vi "AlliGator Menu Items.vi"(8 "Error In":errorcluster, 9 "Menu Item Tag":string, 11 "This VI":refnum<vi>) -> (0 "Error Out":errorcluster, 1 "Message":string, 2 "Window opened?":bool, 3 "AlliGator Actions":T1[](array[typedef]))   [LabVIEW 2021, in "AlliGator GUI.lvlib"]
doc: "Handles AlliGator menu items that are always responsive, including when AlliGator is busy."
uses:
  AlliGator GUI.lvlib
  Action Engine/AlliGator Q Element.ctl
  Action Engine/AlliGator Q Event.ctl
  AlliGator Windows List.ctl
  AlliGator Open Wndow Event Data.ctl
  GUI/Open VI Options.ctl
  Globals, Variables, Constants/AlliGator Variables List.ctl
  Intensity Corrections/AlliGator Define & Save Intensity Corrections File.vi
  Variant/Variant to Data/Variant to Boolean.vi
  Globals, Variables, Constants/AlliGator Abort.vi
  AlliGator Check Version.vi
  <vilib>/Platform/browser.llb/Open URL in Default Browser (string).vi
  Utilities/Utilities.lvlib
  Intensity Corrections/AlliGator Intensity Corrections.lvlib
  Settings/AlliGator Settings.lvlib
  Globals, Variables, Constants/AlliGator Globals, Variables & Constants.lvlib
  Variant/Variant to Data/Variant to Data.lvlib
  Action Engine/AlliGator Action Engine.lvlib
  GUI/GUI.lvlib
panel:
  # "see the AlliGator License on the block diagram (Ctrl+E or Window:Show Block Diagram)"
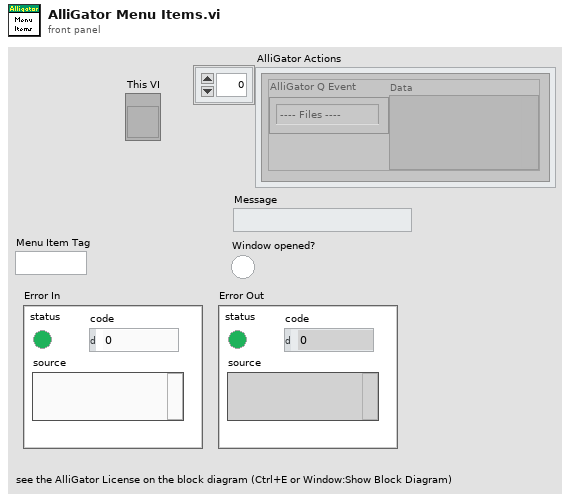
[diagram p1: front panel]
types:
  T1 = typedef "AlliGator Action Engine.lvlib/AlliGator Q Element.ctl" = cluster{"AlliGator Q Event":T2, "Data":variant}
  T2 = typedef "AlliGator Action Engine.lvlib/AlliGator Q Event.ctl" = enum16{"---- Files ----", "Files:Set Batch Export Files To Save", "Files:Set Dataset Loading & Pre-processing Options", "Files:Check #Frames in Dataset", "Files:Increment Frame Index", "Files:Open Mask Image", "Files:Open White Light Image", "Files:Open Single Dataset", "Files:New Folder of Folders Selected", "Files:Load File (all Types)_Scriptable", "Files:Move Flattened Series to Folders Series", "Files:Select Folder", "Files:Load FLI Dataset", "Files:Load Swiss SPAD 1 Dataset", "Files:Load Swiss SPAD 2 Dataset", "Files:Load .sdt FLI Dataset", "Files:Load .ptu FLI Dataset", "Files:Load .bin FLI Dataset", "Files:Load Single Gate Image Folder", "Files:Load I/m/phi Dataset (deprecated)", "Files:Load Single Image", "Files:Subtract Background File", "Files:Export FLI Dataset", "Files:Load HDF5 FLI Dataset", "Files:Set Destination File Path", "Files:Save Mask Image", "Files:Batch Conversion", "Files:New Folder Selected", "Files:Close FLI Dataset", "Files:Close FLI Dataset Series", "Files:Close White Light Image", "Files:Close Mask Image", "---- FLI Dataset ----", "FLI Dataset:Channel Arithmetic", "FLI Dataset:Export Average Lifetime Map as ASCII", "FLI Dataset:Export User-Defined Quantity Map as ASCII", "FLI Dataset:Python Function FLI Dataset Event", "FLI Dataset:ROI Analysis", "FLI Dataset:Tilted Logistic Square Gated IRF Characteristics Map", "FLI Dataset:Logistic Square Gated IRF Characteristics Map", "FLI Dataset:Square Gated IRF Characteristics Map", "FLI Dataset:Multi-ROI Single-Pixel Phasor Analysis", "FLI Dataset:Multi-ROI Single-Pixel NLSF Analysis", "FLI Dataset:All ROIs IRF Extraction", "FLI Dataset:All ROIs Decay Fit Non-Interactive (Fast + Individual IRF)", "FLI Dataset:All ROIs Phasor Analysis", "FLI Dataset:All ROIs Decay Fit", "FLI Dataset:Fluorescence Decay Statistics", "FLI Dataset:Update Decay Statistics Graph", "FLI Dataset:Get Decay from ROI", "FLI Dataset:All ROIs Average Lifetimes", "---- FLI Dataset Series ----", "FLI Dataset Series:Sum All Datasets in Series", "FLI Dataset Series:Add Dataset to Accumulated Dataset", "FLI Dataset Series:Display Accumulated Dataset", "FLI Dataset Series:Clear Dataset Series Sum", "FLI Dataset Series:Time-Series Analysis (NLSF)", "FLI Dataset Series:Time-Series Analysis (Phasor)", "---- Image ----", "Image:Update Image Profile Plots", "Image:Image Histogram Cursor Move", "Image:Image Histogram", "Image:Image Contrast", "Image:Set Image Histogram Cursor Move Flag", "Image:Clear Image Overlay", "Image:Use ROI as Search Area", "Image:Set ROI Diameter", "Image:Save Image Data as TIFF", "Image:Save Displayed Image with Overlay", "Image:Save Image Overlay Only", "Image:Save Image as Hot Pixel Mask", "Image:Change Source Image Color Palette", "Image:Copy Image to Clipboard", "Image:Source Image ROI Selection", "Image:Delete All ROIs", "Image:Delete All Unselected ROIs", "Image:Delete ROI", "Image:Merge All ROIs", "Image:Store ROI", "Image:Source Image ROI Storage", "Image:Export ROI Description to Notebook", "Image:Save ROI", "Image:Load ROI", "Image:Paste ROI Definition", "Image:Clear ROI", "Image:Identify ROIs in Mask Image", "Image:Create Complementary ROI", "Image:Create Contour ROI", "Image:Create ROI(s) from Pixels with Peak above Min_Scriptable", "Image:Create ROI(s) from Pixels with Intensity above Min_Scriptable", "Image:Compute ROI Statistics", "Image:Delete ROI(s) based on ROI Characteristics", "Image:Create ROI Grid", "Image:ROI to Individual Pixel ROIs", "Image:Python Function Source Image Event", "Image:Show Phasor Calibration Map ROI Centers", "Image:Convert ROI to Mask Image", "Image:Mouse Move", "Image:Mouse Up", "Image:Set Source Image Mouse Move Flag", "Image:Add Scale Bar Overlay", "Image:Delete Existing ROIs Option", "Image:Overlay ROI Median", "Image:Check Current ROI", "---- Decay ----", "Decay:Clear IRF/Reference Plot", "Decay:Clear Local IRFs", "Decay:Add Decay to Graph", "Decay:Smoothen Plot", "Decay:Smoothen Plot Tail", "Decay:Average Selected Plots", "Decay:Extract IRF", "Decay:Optimal IRF Extraction", "Decay:Threshold IRF", "Decay:Fit to Model IRF", "Decay:Fit IRF to Square Gate", "Decay:Fit IRF to Logistic Square Gate", "Decay:Fit IRF to Tilted Logistic Square Gate", "Decay:Create Bounding Cursors Set", "Decay:Export Bounding Cursors Definition to Notebook", "Decay:Denoise Plot", "Decay:Compute Cumulative Function", "Decay:Use as Reference Decay", "Decay:Show Reference Decay/IRF", "Decay:Extrapolate Decay", "Decay:Create Head & Tail Bounding Cursors", "Decay:Store Cursor-defined Head & Tail Fractions", "Decay:Rebin Plot", "Decay:1-Normalize Decay", "Decay:[0-1]-Normalize Plot", "Decay:Straighten Decay", "Decay:Shift Decay", "Decay:Fold Decay", "Decay:Fit Decay", "Decay:Global Fit of Selected Decays", "Decay:Post Global Fit Script", "Decay:Add Global Fit Parameters to Graph", "Decay:Add Decay Parameter(s) to Plot (Graph)", "Decay:Export Decay to Phasor Graph", "Decay:Plot Decay Shifts", "Decay:Compute Average Lifetime", "Decay:Plot Convolution", "Decay:Graph Tip Strip Update", "---- Decay Statistics ----", "Decay Statistics:Tip Strip Update", "---- Intensity Time Trace ----", "Intensity Time Trace:Use File Timestamp", "Intensity Time Trace:Load Intensity Corrections File", "Intensity Time Trace:Clear Intensity Corrections File", "Intensity Time Trace:Tip Strip Update", "---- Phasor Plot ----", "Phasor Plot:Build Phasor Plot", "Phasor Plot:Change Phasor Plot Color Palette", "Phasor Plot:Adjust Phasor Plot Display Range", "Phasor Plot:Highlight Image ROI in Phasor Plot", "Phasor Plot:Save Phasor Plot Image with Overlay", "Phasor Plot:Export Complex Phasor Map", "Phasor Plot:Export Phasor Ratio Map", "Phasor Plot:Export Average Lifetime Map", "Phasor Plot:Compute Phase Lifetime Histogram", "Phasor Plot:Compute Phasor Ratio Histogram", "Phasor Plot:Compute Phase Lifetime vs Intensity Scatter Plot", "Phasor Plot:Weber 2-Component Decomposition", "Phasor Plot:Update Phasor Color Map Vertices", "Phasor Plot:Clear Phasor Overlay", "Phasor Plot:Use Segment Extremities as References", "Phasor Plot:Use UC/Segment Intersections as References", "Phasor Plot:Use UC/Principal Axis Intersections as References", "Phasor Plot:Use UC/Linear Fit Intersections as References", "Phasor Plot:Update Phasor Plot Reference", "Phasor Plot:Show Local Phasor Info in Phasor Plot", "Phasor Plot:Update Phasor Plot State", "Phasor Plot:Phasor Plot ROI Storage", "Phasor Plot:Phasor Plot ROI Selection", "Phasor Plot:Python Function Phasor Plot Event", "Phasor Plot:Overlay Phasor ROI, Ratio or Map in Source Image", "Phasor Plot:Compute Decay of Selected Phasors", "Phasor Plot:Phasor at Image Pixel", "Phasor Plot:Mouse Move", "Phasor Plot:Mouse Up", "Phasor Plot:Display Range Mouse Move", "Phasor Plot:Set Mouse Move Flag", "---- Phasor Graph ----", "Phasor Graph:Calibrated Phasor Map Series", "Phasor Graph:Whole Image Phasor Scatter Plot (deprecated)", "Phasor Graph:Get Phasor Value", "Phasor Graph:Create New Phasor Plot Dialog", "Phasor Graph:Update Last Phasor Value", "Phasor Graph:Update Phasor (m, phi)", "Phasor Graph:Remove Single Phasor from Plot", "Phasor Graph:Add Single Phasor to Plot", "Phasor Graph:Remove Phasor Plot", "Phasor Graph:Remove Selected Phasor Plots", "Phasor Graph:Clear Phasor Data", "Phasor Graph:Clear Phasor Graph", "Phasor Graph:Cursor Move", "Phasor Graph:Draw Cursor Connecting Line", "Phasor Graph:Clear Cursor Connecting Line", "Phasor Graph:Find UC Intersection", "Phasor Graph:Use UC/Cursor-Defined Line Intersections", "Phasor Graph:Use Selected Plots Fitted Line/UC Intersections", "Phasor Graph:Use Selected Plots Principal Axis/UC Intersections", "Phasor Graph:Show Single Phasor", "Phasor Graph:Save Single Phasor Plot", "Phasor Graph:Save All Phasor Plots", "Phasor Graph:Load Phasor Plot(s)", "Phasor Graph:Phasor Multiplication", "Phasor Graph:Compute Average Phasor", "Phasor Graph:Compute Multiple Average Phasors (Selected Plots)", "Phasor Graph:Export Single Phasor Plot Phase Lifetimes", "Phasor Graph:Phase Lifetime Trajectory", "Phasor Graph:Phase Lifetime vs Intensity Scatter Plot (deprecated)", "Phasor Graph:Parameter 2 vs Parameter 1 Scatter Plot", "Phasor Graph:Use Cursor n Location", "Phasor Graph:Set Reference n to Current Phase Lifetime Value", "Phasor Graph:Set Reference n to Lifetime Value", "Phasor Graph:Set Cursor n Location", "Phasor Graph:Save Phasor Graph Image", "Phasor Graph:Update SEPL Plot", "Phasor Graph:Export Single Phasor Plot Data", "Phasor Graph:Export Selected Phasor Plots Data", "Phasor Graph:Python Function Phasor Graph Event", "Phasor Graph:Tip Strip Update", "---- Calibration ----", "Calibration:Set Calibration Type", "Calibration:Load/Save Phasor Calibration", "Calibration:Load/Save Phasor Calibration Series", "Calibration:Load/Save Phasor Calibration Map", "Calibration:Use as Calibration", "Calibration:Compute Optimal Calibration from Phasor References", "Calibration:Clear Phasor Calibration", "Calibration:Single Phasor Calibration Information", "Calibration:Use as Calibration Series", "Calibration:Use as Calibration Map", "Calibration:Clear Calibration Series", "Calibration:Phasor Calibration Series Information", "Calibration:Clear Calibration Map", "Calibration:Phasor Calibration Map Information", "Calibration:Apply Phasor Calibration", "Calibration:Update Single Plot Calibration", "Calibration:Update Multiple Plots Calibration", "Calibration:Clear Single Plot Calibration", "Calibration:Clear All Plots Calibrations", "Calibration:Clear Plot(s) Calibration(s)?", "Calibration:Phasor Calibration Maps (# Gates Series)", "---- Phasor Ratio ----", "Phasor Ratio:Clear Reference n", "Phasor Ratio:Toggle Selected Plot(s)  Lock to Reference 1", "Phasor Ratio:Use as Reference n", "Phasor Ratio:Send Reference n to Notebook", "Phasor Ratio:Toggle Selected Plot(s)  Lock to Reference 2", "Phasor Ratio:Compute Phasor Ratio at Mouse Location", "Phasor Ratio:Compute Phasor Plot's Average Phasor Ratio", "Phasor Ratio:Compute Time-Series Phasor Ratios", "Phasor Ratio:Fit Line to Phasor Ratio Plot", "Phasor Ratio:Save References", "Phasor Ratio:Load References", "Phasor Ratio:Update Phasor Reference 1", "Phasor Ratio:Update Phasor Reference 2", "Phasor Ratio:Move Cursor n to Reference n", "Phasor Ratio:Use as Phasor Reference 1 Lifetime", "Phasor Ratio:Use as Phasor Reference 2 Lifetime", "Phasor Ratio:Export Phasor Ratio Map as ASCII", "Phasor Ratio:Tip Strip Update", "---- Lifetime & Other Parameters Graph ----", "Lifetime:Tip Strip Update", "---- Decay Fit Parameter Map ----", "Decay Fit Parameter Map:Export ROI NLSF Data as ASCII", "Decay Fit Parameter Map:Set Decay Fit Parameter Map Selection", "Decay Fit Parameter Map:Build Decay Fit Parameter Map", "Decay Fit Parameter Map:Change Decay Fit Parameter Map Color Palette", "Decay Fit Parameter Map:Export Decay Fit Parameter Map Data as ASCII", "Decay Fit Parameter Map:Export All Decay Fit Parameter Maps Data as ASCII", "Decay Fit Parameter Map:Selected Parameter Scatterplot", "Decay Fit Parameter Map:Parameter 2 vs Parameter 1 Scatterplot", "Decay Fit Parameter Map:Save Decay Fit Parameter Map Image", "Decay Fit Parameter Map:Save-Load IRFs & Fit Data", "Decay Fit Parameter Map:Update Local Decay Plots", "Decay Fit Parameter Map:Python Function Decay Fit Parameters Map Event", "Decay Fit Parameter Map:Overlay Decay Fit Parameter Map in Source Image", "Decay Fit Parameter Map:Selected Parameter vs Intensity Scatterplot", "Decay Fit Parameter Map:Mouse Up", "Decay Fit Parameter Map:Display Range Mouse Move", "---- Parameter Map ----", "Parameter Map:Export ROI Parameters Data as ASCII", "Parameter Map:Delete Parameter Map Set", "Parameter Map:Update Parameter List", "Parameter Map:Build Parameter Map", "Parameter Map:Change Parameter Map Color Palette", "Parameter Map:Export Parameter Map Data as ASCII", "Parameter Map:Export All Parameter Maps Data as ASCII", "Parameter Map:Selected Parameter Scatterplot", "Parameter Map:Parameter 2 vs Parameter 1 Scatterplot", "Parameter Map:Selected Parameter vs Intensity Scatterplot", "Parameter Map:Save Parameter Map Image", "Parameter Map:Save-Load IRFs & Parameter Maps (TODO)", "Parameter Map:Set Parameter Map Selection", "Parameter Map:Python Function Parameter Map Event", "Parameter Map:Overlay Parameter Map in Source Image", "Parameter Map:Update Local Decay Plots", "Parameter Map:Mouse Up", "Parameter Map:Display Range Mouse Move", "---- Generic Graph ----", "Generic Graph:Generic XY Graph Event", "Generic Graph:Python Function XY Graph Event", "Generic Graph:New Plot", "Generic Graph:Save Plot", "Generic Graph:XY Plot Histogram", "Generic Graph:Set XY Graph Plot Name", "Generic Graph:Set Last Cursor Style", "Generic Graph:Tip Strip Update", "---- GUI ----", "GUI:Start Script", "GUI:Type of Displayed Image Changed", "GUI:Gate Image Slide Changed", "GUI:Show Busy Icon", "GUI:Show Busy Icon & Abort Button", "GUI:Hide Busy Icon", "GUI:Hide Busy Icon & Abort Button", "GUI:Abort", "GUI:End Script", "GUI:Start Timing", "GUI:End Timing", "GUI:Set State Indicator", "GUI:Send Parameters JSON Strings to Clipboard", "GUI:Set Gate Step", "GUI:Idle", "GUI:Initialization", "GUI:Quit", "GUI:Increment Dataset Index", "GUI:Set Dataset Index to -1", "GUI:Time Series Slider Moved", "GUI:Time Series Slider Changed", "GUI:Toggle Playback or Loop", "GUI:Playback Script", "GUI:Set Phasor Frequency", "GUI:Open Window", "GUI:Start Test Script", "GUI:End Test Script", "DEBUG"}
  T3 = typedef "AlliGator GUI.lvlib/AlliGator Open Wndow Event Data.ctl" = cluster{"AlliGator Windows":T4, "Open Window Options":T5}
  T4 = typedef "AlliGator GUI.lvlib/AlliGator Windows List.ctl" = enum16{"AlliGator Window", "Settings Window", "Notebook Window", "Dataset Information Window", "Source Image ROI Manager Window", "Phasor Plot ROI Manager Window", "Phasor Harmonic Manager Window", "Histogram Window", "Image Profile Window", "Local Decay Window", "About Window", "Batch Conversion Window", "Shot Noise Influence on Average Lifetime", "Fit Method Benchmark", "AlliGator Alias Definition"}
  T5 = typedef "GUI.lvlib/Open VI Options.ctl" = cluster{"Bring To Front (T)":bool, "Start Hidden? (F)":bool, "Activate? (T)":bool}
  T6 = typedef "AlliGator Globals, Variables & Constants.lvlib/AlliGator Variables List.ctl" = enum16{"---- GUI ----", "GUI:Initialization Status", "GUI:State Indicators Refnum", "GUI:Original AlliGator Menu Items", "GUI:Current Action Loop State", "GUI:Script in progress", "GUI:Playback", "GUI:Loop Playback", "GUI:Search ROI Used", "GUI:Search ROI", "Decay Graph Max Legend Size", "Intensity Graph Max Legend Size", "Decay Statistics Graph Max Legend Size", "Phasor Graph Max Legend Size", "Phasor Ratio Graph Max Legend Size", "Lifetime Graph Max Legend Size", "---- Files ----", "Files:Export Dataset Frames as Individual Files", "Files:Show Batch Export Help Balloons", "Files:Frames in Dataset", "Files:ptu File Frame Start Indices", "Files:Current Frame in Dataset", "Files:Current Frame Timestamp", "Files:Dataset Loaded", "Files:Dataset Metadata", "Files:Dataset Channel", "Files:Dataset Data Description", "Files:Background Dataset Metadata", "Files:Background Dataset Channel", "Files:Background Dataset Data Description", "Files:Background File Subtraction", "Files:Background File Path", "Files:Background File Pile-up Correction", "Files:Background File Pixel Well Capacity", "Files:Background File Scaling Factor", "Files:Current Dataset Load Settings", "Files:Dataset Path", "Files:ICCD-specific Information", "Files:Macrotime Gate Separation", "------ Python Plugins ------", "Python Plugins:Information", "Python Plugins:Python Session", "Python Plugins:Valid Python Session?", "---- Source Image ----", "Source Image:ROIs", "Source Image:Current ROI", "Source Image:ROI Event Refnum", "X_Source Image Display Range", "X_Source Image Palette Information", "X_Type of Displayed Image", "X_Time Gate Slider", "Source Image:Palette List", "Source Image:Scale", "Source Image:ROI Overlay Color", "Source Image:Overlay to Erase", "Source Image:Is Displayed Image Accumulated", "Source Image:White Light Image Modified", "Source Image:Mask Image Modified", "---- Image Profile Window ----", "Image Profile:Window Event Refnum", "Image Profile:IntensityType", "Image Profile:Intensity Average Type", "Image Profile:Intensity-weighted SDV", "Image Profile:Box Profile Type", "Image Profile:Window Open", "Image Profile:Plotted Fit Parameter", "------ Phasor Graph -------", "Phasor Graph:Show Line", "---- Phasor Plot ---", "Phasor Plot:Parameters Changed", "Phasor Plot:FLI Dataset Modified since last Calculation", "Phasor Harmonics Data", "Selected Phasor Harmonics", "Phasor Harmonic Manager Event Refnum", "Phasor Plot:ROIs", "Phasor Plot:Current ROI", "Phasor Plot:ROI Event Refnum", "Phasor Plot:Image Reference Points", "Phasor Plot:Computed", "Phasor Plot:Palette Information", "Phasor Plot:Palette List", "Phasor Plot:Phasor Ratio Palette Information", "Phasor Plot:Phasor Ratio Palette List", "Phasor Plot:Image Scale", "Phasor Plot:Image Overlay to Erase", "Phasor Plot:Image Elements to Update", "Phasor Plot:Current Calculation Parameters", "Phasor Plot:Current Calibration Options", "Phasor Plot:Reset Cumulated Phasor Plot", "Phasor Plot:Reference 1", "Phasor Plot:Lifetime Reference 1", "Phasor Plot:Reference 1 Frequency", "Phasor Plot:Reference 2", "Phasor Plot:Lifetime Reference 2", "Phasor Plot:Reference 2 Frequency", "---- Decay Analysis ----", "Number of Selected Decays to Fit", "LS Fit Results", "LAR Fit Results", "BS Fit Results", "Last Decay Max - Min", "Best Fit Parameters", "Best Fit Parameter Names", "Actual Size X", "Actual Size Y", "Binning X", "Binning Y", "Actual # Gates", "Dataset Number", "Gates to...", "Gates Skipped", "Gates to keep", "Gate Step", "Gate Separation", "Reversed Gates", "Pile-up Correction", "Pixel Well Capacity", "Background Subtracted", "Background Subtraction Method", "Background Definition Range", "Background File (deprecated)", "Number of Dataset Accumulated", "Array of Accumulated Dataset Paths", "Do Averaged Datasets", "Destination File Path", "Process Plot Target", "Use 1/D as Phasor Frequency", "---- Decay Fit Parameter Map -----", "Decay Fit Parameter Map:Palette Information", "Decay Fit Parameter Map:Palette List", "---- Parameter Map ----", "Parameter Map:Palette Information", "Parameter Map:Palette List", "------- Local Decay Window ---------", "Local Decay Graph Window:Event Refnum", "Local Decay Graph Window:Use normalized IRF for convolution", "----- Miscellaneous ----", "Misc:Skippable Dialog Windows Status"}
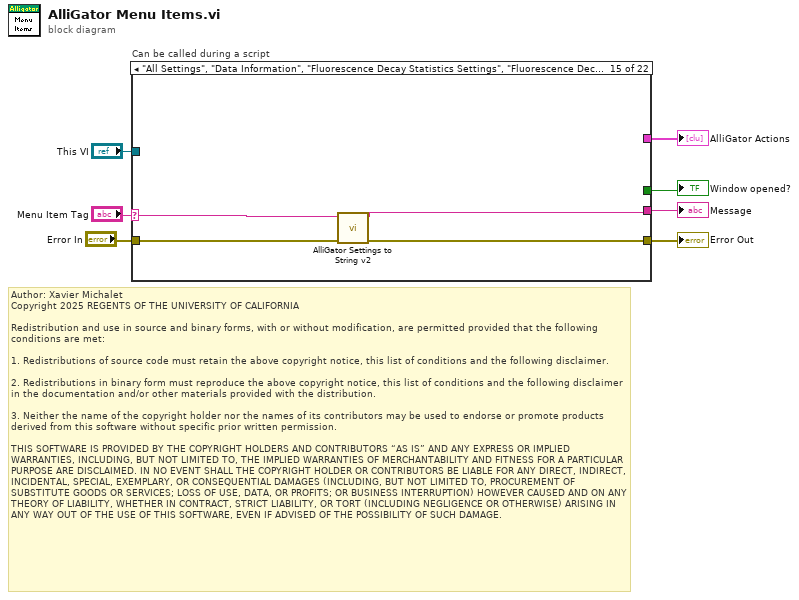
[diagram p0: block diagram]
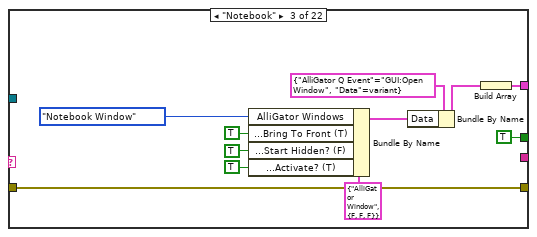
[diagram p4: hidden frame]
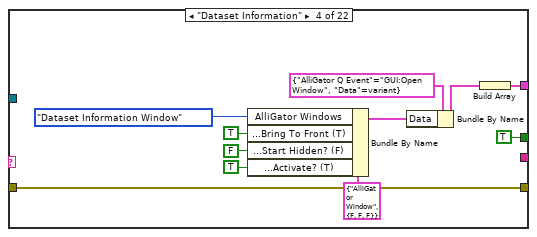
[diagram p5: hidden frame]
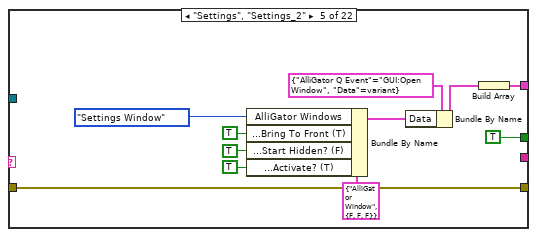
[diagram p6: hidden frame]
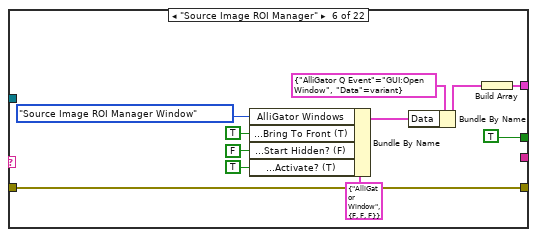
[diagram p7: hidden frame]
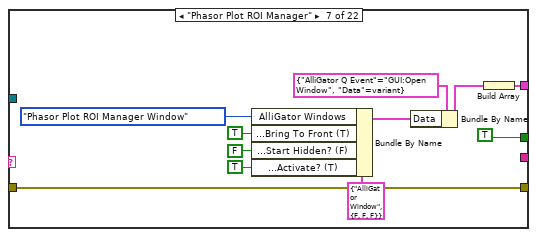
[diagram p8: hidden frame]
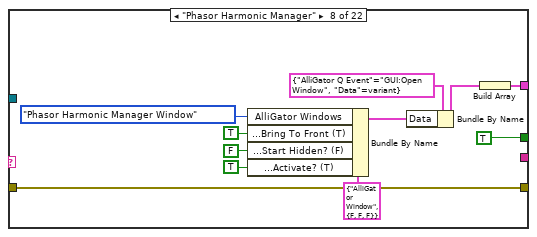
[diagram p9: hidden frame]
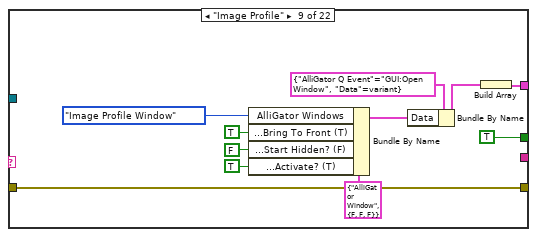
[diagram p10: hidden frame]
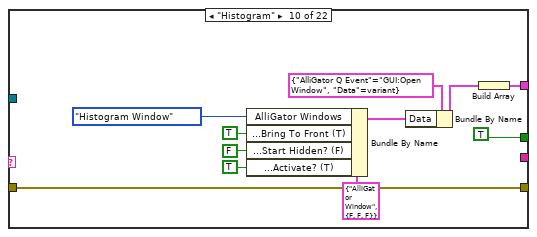
[diagram p11: hidden frame]
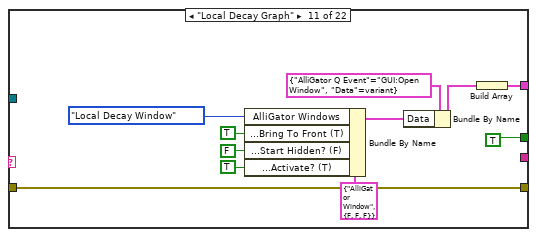
[diagram p12: hidden frame]
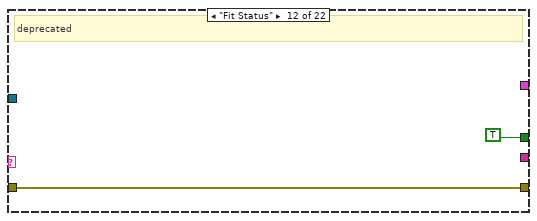
[diagram p13: hidden frame]
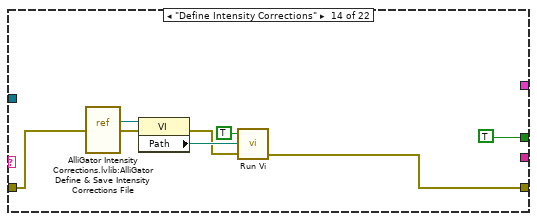
[diagram p15: hidden frame]
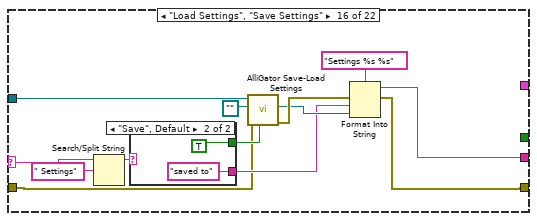
[diagram p16: hidden frame]
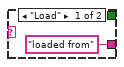
[diagram p17: hidden frame]
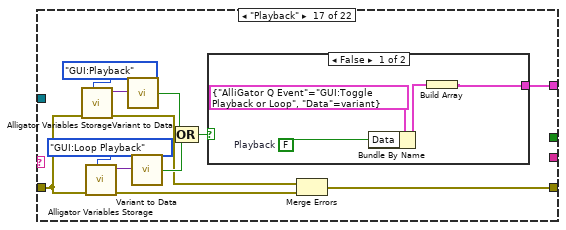
[diagram p18: hidden frame]
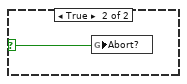
[diagram p19: hidden frame]
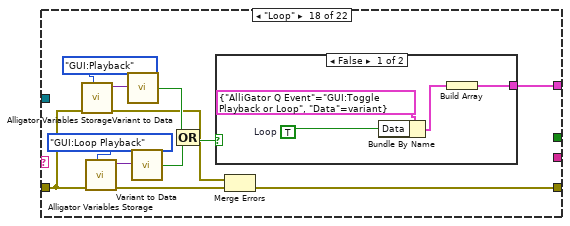
[diagram p20: hidden frame]
diagram:
  # "Author: Xavier Michalet\nCopyright 2025 REGENTS OF THE UNIVERSITY OF CALIFORNIA\n\nRedistribution and use in source and binary forms, with or without modification, are permitted provided that the following conditions are met:\n\n1. Redistributions of source code must retain the above copyright notice, this list of conditions and the following disclaimer.\n\n2. Redistributions in binary form must reproduce the above copyright notice, this list of conditions and the following disclaimer in the documentation and/or other materials provided with the distribution.\n\n3. Neither the name of the copyright holder nor the names of its contributors may be used to endorse or promote products derived from this software without specific prior written permission.\n\nTHIS SOFTWARE IS PROVIDED BY THE COPYRIGHT HOLDERS AND CONTRIBUTORS “AS IS” AND ANY EXPRESS OR IMPLIED WARRANTIES, INCLUDING, BUT NOT LIMITED TO, THE IMPLIED WARRANTIES OF MERCHANTABILITY AND FITNESS FOR A PARTICULAR PURPOSE ARE DISCLAIMED. IN NO EVENT SHALL THE COPYRIGHT HOLDER OR CONTRIBUTORS BE LIABLE FOR ANY DIRECT, INDIRECT, INCIDENTAL, SPECIAL, EXEMPLARY, OR CONSEQUENTIAL DAMAGES (INCLUDING, BUT NOT LIMITED TO, PROCUREMENT OF SUBSTITUTE GOODS OR SERVICES; LOSS OF USE, DATA, OR PROFITS; OR BUSINESS INTERRUPTION) HOWEVER CAUSED AND ON ANY THEORY OF LIABILITY, WHETHER IN CONTRACT, STRICT LIABILITY, OR TORT (INCLUDING NEGLIGENCE OR OTHERWISE) ARISING IN ANY WAY OUT OF THE USE OF THIS SOFTWARE, EVEN IF ADVISED OF THE POSSIBILITY OF SUCH DAMAGE."
  n1 = case "Can be called during a script" shown="\"All Settings\", \"Data Information\", \"Fluorescence Decay Statistics Settings\", \"Fluorescence Decay_Advanced Analysis\", \"Fluorescence Decay_All\", \"Fluorescence Decay_Decay Pre-Processing\", \"Fluorescence Decay_Fit Options\", \"Fluorescence Decay_Fit Parameters\", \"Fluorescence Decay_Styles\", \"Intensity Time Trace Settings\", \"Lifetime Analysis Settings\", \"Miscellaneous Settings\", \"Phasor Graph Settings\", \"Phasor Plot Settings\", \"Single-Exponential Phasor Locus (SEPL) Settings\", \"Source Image Settings\"" "Menu Item Tag" {
    selector: "Menu Item Tag" -> [_ _ _ _ _ _ _ _ _ _ _ _ _ _ w122 w131 _ _ _ _ _ _]
    tunnel: "This VI" -> [_ _ _ _ _ _ _ _ _ _ _ _ _ _ _ w135 _ _ _ _ _ _]
    tunnel: [_ _ w15 w23 w34 w45 w56 w67 w78 w89 w100 _ _ _ _ _ w143 w160 _ w176 _ _] -> w2
    tunnel: [_ _ _ _ _ _ _ _ _ _ _ _ _ _ w121 w125 _ _ _ _ _ _] -> w5
    tunnel: "Error In" -> [w8 w9 w10 w21 w32 w43 w54 w65 w76 w87 w98 w109 w111 w113 w120 w123 w142 w159 w173 w174 w190 w196]
    tunnel: [w8 w9 w10 w21 w32 w43 w54 w65 w76 w87 w98 w109 w111 w114 w119 w124 w140 w157 w173 w174 w191 w197] -> w3
    tunnel: [_ _ TRUE ("Start Hidden? (F)") TRUE ("Start Hidden? (F)") TRUE ("Start Hidden? (F)") TRUE ("Start Hidden? (F)") TRUE ("Start Hidden? (F)") TRUE ("Start Hidden? (F)") TRUE ("Start Hidden? (F)") TRUE ("Start Hidden? (F)") TRUE ("Start Hidden? (F)") TRUE ("Start Hidden? (F)") _ TRUE ("Start Hidden? (F)") _ _ _ _ _ TRUE ("Start Hidden? (F)") TRUE ("Start Hidden? (F)") _] -> w1
    frame "", Default {
    }
    frame "---- Windows ----" {
    }
    frame "Notebook" {
      n2 = Bundle By Name(cluster=T3 {"AlliGator Windows"=enum."AlliGator Window", "Open Window Options"={"Bring To Front (T)"=FALSE, "Start Hidden? (F)"=FALSE, "Activate? (T)"=FALSE}} ("output cluster"), "AlliGator Windows"=AlliGator_Windows_List."Notebook Window", "Open Window Options.Bring To Front (T)"=TRUE, "Open Window Options.Start Hidden? (F)"=TRUE ("Start Hidden? (F)"), "Open Window Options.Activate? (T)"=TRUE) -> (w19:T3)
      n3 = Bundle By Name(cluster=T1 {"AlliGator Q Event"=enum."GUI:Open Window", "Data"=variant}, "Data"=w19) -> (w18:T1)
      n4 = Build Array(w18) -> (w15:T1[])
    }
    frame "Dataset Information" {
      n5 = Bundle By Name(cluster=T3 {"AlliGator Windows"=enum."AlliGator Window", "Open Window Options"={"Bring To Front (T)"=FALSE, "Start Hidden? (F)"=FALSE, "Activate? (T)"=FALSE}} ("output cluster"), "AlliGator Windows"=AlliGator_Windows_List."Dataset Information Window", "Open Window Options.Bring To Front (T)"=TRUE, "Open Window Options.Start Hidden? (F)"=FALSE ("Start Hidden? (F)"), "Open Window Options.Activate? (T)"=TRUE) -> (w30:T3)
      n6 = Bundle By Name(cluster=T1 {"AlliGator Q Event"=enum."GUI:Open Window", "Data"=variant}, "Data"=w30) -> (w29:T1)
      n7 = Build Array(w29) -> (w23:T1[])
    }
    frame "Settings", "Settings_2" {
      n8 = Bundle By Name(cluster=T3 {"AlliGator Windows"=enum."AlliGator Window", "Open Window Options"={"Bring To Front (T)"=FALSE, "Start Hidden? (F)"=FALSE, "Activate? (T)"=FALSE}} ("output cluster"), "AlliGator Windows"=AlliGator_Windows_List."Settings Window", "Open Window Options.Bring To Front (T)"=TRUE, "Open Window Options.Start Hidden? (F)"=TRUE ("Start Hidden? (F)"), "Open Window Options.Activate? (T)"=TRUE) -> (w41:T3)
      n9 = Bundle By Name(cluster=T1 {"AlliGator Q Event"=enum."GUI:Open Window", "Data"=variant}, "Data"=w41) -> (w40:T1)
      n10 = Build Array(w40) -> (w34:T1[])
    }
    frame "Source Image ROI Manager" {
      n11 = Bundle By Name(cluster=T3 {"AlliGator Windows"=enum."AlliGator Window", "Open Window Options"={"Bring To Front (T)"=FALSE, "Start Hidden? (F)"=FALSE, "Activate? (T)"=FALSE}} ("output cluster"), "AlliGator Windows"=AlliGator_Windows_List."Source Image ROI Manager Window", "Open Window Options.Bring To Front (T)"=TRUE, "Open Window Options.Start Hidden? (F)"=FALSE ("Start Hidden? (F)"), "Open Window Options.Activate? (T)"=TRUE) -> (w52:T3)
      n12 = Bundle By Name(cluster=T1 {"AlliGator Q Event"=enum."GUI:Open Window", "Data"=variant}, "Data"=w52) -> (w51:T1)
      n13 = Build Array(w51) -> (w45:T1[])
    }
    frame "Phasor Plot ROI Manager" {
      n14 = Bundle By Name(cluster=T3 {"AlliGator Windows"=enum."AlliGator Window", "Open Window Options"={"Bring To Front (T)"=FALSE, "Start Hidden? (F)"=FALSE, "Activate? (T)"=FALSE}} ("output cluster"), "AlliGator Windows"=AlliGator_Windows_List."Phasor Plot ROI Manager Window", "Open Window Options.Bring To Front (T)"=TRUE, "Open Window Options.Start Hidden? (F)"=FALSE ("Start Hidden? (F)"), "Open Window Options.Activate? (T)"=TRUE) -> (w63:T3)
      n15 = Bundle By Name(cluster=T1 {"AlliGator Q Event"=enum."GUI:Open Window", "Data"=variant}, "Data"=w63) -> (w62:T1)
      n16 = Build Array(w62) -> (w56:T1[])
    }
    frame "Phasor Harmonic Manager" {
      n17 = Bundle By Name(cluster=T3 {"AlliGator Windows"=enum."AlliGator Window", "Open Window Options"={"Bring To Front (T)"=FALSE, "Start Hidden? (F)"=FALSE, "Activate? (T)"=FALSE}} ("output cluster"), "AlliGator Windows"=AlliGator_Windows_List."Phasor Harmonic Manager Window", "Open Window Options.Bring To Front (T)"=TRUE, "Open Window Options.Start Hidden? (F)"=FALSE ("Start Hidden? (F)"), "Open Window Options.Activate? (T)"=TRUE) -> (w74:T3)
      n18 = Bundle By Name(cluster=T1 {"AlliGator Q Event"=enum."GUI:Open Window", "Data"=variant}, "Data"=w74) -> (w73:T1)
      n19 = Build Array(w73) -> (w67:T1[])
    }
    frame "Image Profile" {
      n20 = Bundle By Name(cluster=T3 {"AlliGator Windows"=enum."AlliGator Window", "Open Window Options"={"Bring To Front (T)"=FALSE, "Start Hidden? (F)"=FALSE, "Activate? (T)"=FALSE}} ("output cluster"), "AlliGator Windows"=AlliGator_Windows_List."Image Profile Window", "Open Window Options.Bring To Front (T)"=TRUE, "Open Window Options.Start Hidden? (F)"=FALSE ("Start Hidden? (F)"), "Open Window Options.Activate? (T)"=TRUE) -> (w85:T3)
      n21 = Bundle By Name(cluster=T1 {"AlliGator Q Event"=enum."GUI:Open Window", "Data"=variant}, "Data"=w85) -> (w84:T1)
      n22 = Build Array(w84) -> (w78:T1[])
    }
    frame "Histogram" {
      n23 = Bundle By Name(cluster=T3 {"AlliGator Windows"=enum."AlliGator Window", "Open Window Options"={"Bring To Front (T)"=FALSE, "Start Hidden? (F)"=FALSE, "Activate? (T)"=FALSE}} ("output cluster"), "AlliGator Windows"=AlliGator_Windows_List."Histogram Window", "Open Window Options.Bring To Front (T)"=TRUE, "Open Window Options.Start Hidden? (F)"=FALSE ("Start Hidden? (F)"), "Open Window Options.Activate? (T)"=TRUE) -> (w96:T3)
      n24 = Bundle By Name(cluster=T1 {"AlliGator Q Event"=enum."GUI:Open Window", "Data"=variant}, "Data"=w96) -> (w95:T1)
      n25 = Build Array(w95) -> (w89:T1[])
    }
    frame "Local Decay Graph" {
      n26 = Bundle By Name(cluster=T3 {"AlliGator Windows"=enum."AlliGator Window", "Open Window Options"={"Bring To Front (T)"=FALSE, "Start Hidden? (F)"=FALSE, "Activate? (T)"=FALSE}} ("output cluster"), "AlliGator Windows"=AlliGator_Windows_List."Local Decay Window", "Open Window Options.Bring To Front (T)"=TRUE, "Open Window Options.Start Hidden? (F)"=FALSE ("Start Hidden? (F)"), "Open Window Options.Activate? (T)"=TRUE) -> (w107:T3)
      n27 = Bundle By Name(cluster=T1 {"AlliGator Q Event"=enum."GUI:Open Window", "Data"=variant}, "Data"=w107) -> (w106:T1)
      n28 = Build Array(w106) -> (w100:T1[])
    }
    frame "Fit Status" {
      # "deprecated"
    }
    frame "---- Analysis ----" {
    }
    frame "Define Intensity Corrections" {
      n29 = vi-ref "AlliGator Intensity Corrections.lvlib:AlliGator Define & Save Intensity Corrections File.vi"() -> (w118:refnum<vi>)
      n30 = property class="VI"(reference=w118, error in=w113) -> (error out=w116:errorcluster, "Path"=w117:path)  [unwired: 1 out]
      n31 = call "Run Vi.vi"("Bring To Front (T)"=TRUE, "VI Path"=w117, "error in (no error)"=w116) -> ("error out"=w114:errorcluster)  [unwired: 5 in, 1 out]
    }
    frame "All Settings", "Data Information", "Fluorescence Decay Statistics Settings", "Fluorescence Decay_Advanced Analysis", "Fluorescence Decay_All", "Fluorescence Decay_Decay Pre-Processing", "Fluorescence Decay_Fit Options", "Fluorescence Decay_Fit Parameters", "Fluorescence Decay_Styles", "Intensity Time Trace Settings", "Lifetime Analysis Settings", "Miscellaneous Settings", "Phasor Graph Settings", "Phasor Plot Settings", "Single-Exponential Phasor Locus (SEPL) Settings", "Source Image Settings" {
      n32 = call "AlliGator Settings to String v2.vi"("error in (no error)"=w120, "Settings to Export (All)"=w122) -> ("error out"=w119:errorcluster, "Message"=w121:string)  [unwired: 8 in]
    }
    frame "Load Settings", "Save Settings" {
      n33 = Search/Split String(string=w131, search string/char (-)=" Settings") -> (substring before match=w129:string)  [unwired: 1 in, 2 out]
      n34 = case shown="\"Save\", Default" w129 {
        tunnel: [_ TRUE ("Load(F)/Save (T)")] -> w134
        tunnel: ["loaded from" ("search string/char (-)") "saved to" ("search string/char (-)")] -> w126
        frame "Load" {
        }
        frame "Save", Default {
        }
      }
      n35 = call "AlliGator Save-Load Settings.vi"("Load(F)/Save (T)"=w134, "Error In"=w123, "File Path"=path "", "AlliGator Refnum in"=w135) -> ("Error Out"=w132:errorcluster, "File Path out"=w127:path)  [unwired: 6 in]
      n36 = Format Into String(format string="Settings %s %s" ("initial string"), error in=w132, w126, w127) -> (resulting string=w125:string, error out=w124:errorcluster)  [unwired: 1 in]
    }
    frame "Playback" {
      n37 = call "Alligator Variables Storage.vi"("AlliGator Variable"=AlliGator_Variables_List."GUI:Playback" ("Alligator Variable"), "Error In"=w142) -> ("Error Out"=w141:errorcluster, "Data out"=w149:variant)  [unwired: 7 in, 1 out]
      n38 = call "Alligator Variables Storage.vi"("AlliGator Variable"=AlliGator_Variables_List."GUI:Loop Playback" ("Alligator Variable"), "Error In"=w142) -> ("Error Out"=w139:errorcluster, "Data out"=w147:variant)  [unwired: 7 in, 1 out]
      n39 = call-poly "Variant to Data.vi"("Variant"=w149) -> ("Value"=w148:bool)  [unwired: 8 in]
      n40 = call-poly "Variant to Data.vi"("Variant"=w147) -> ("Value"=w144:bool)  [unwired: 8 in]
      n41 = Compound Arithmetic op=OR(w148, w144) -> (w145:bool)
      n42 = case shown="False" w145 {
        selector: w145 -> [_ w155]
        tunnel: [w151 _] -> w143
        frame False {
          w152 = FALSE  # Playback
          n43 = Bundle By Name(cluster=T1 {"AlliGator Q Event"=enum."GUI:Toggle Playback or Loop", "Data"=variant} ("element"), "Data"=w152) -> (w153:T1)
          n44 = Build Array(w153) -> (w151:T1[])
        }
        frame True {
          n45 = global write "AlliGator Abort.vi" "Abort?"(w155) -> ()
        }
      }
      n46 = Merge Errors(w141, w139) -> (w140:errorcluster)
    }
    frame "Loop" {
      n47 = call "Alligator Variables Storage.vi"("AlliGator Variable"=AlliGator_Variables_List."GUI:Playback" ("Alligator Variable"), "Error In"=w159) -> ("Error Out"=w156:errorcluster, "Data out"=w166:variant)  [unwired: 7 in, 1 out]
      n48 = call "Alligator Variables Storage.vi"("AlliGator Variable"=AlliGator_Variables_List."GUI:Loop Playback" ("Alligator Variable"), "Error In"=w159) -> ("Error Out"=w158:errorcluster, "Data out"=w164:variant)  [unwired: 7 in, 1 out]
      n49 = call-poly "Variant to Data.vi"("Variant"=w166) -> ("Value"=w165:bool)  [unwired: 8 in]
      n50 = call-poly "Variant to Data.vi"("Variant"=w164) -> ("Value"=w162:bool)  [unwired: 8 in]
      n51 = Compound Arithmetic op=OR(w165, w162) -> (w161:bool)
      n52 = case shown="False" w161 {
        selector: w161 -> [_ w172]
        tunnel: [w168 _] -> w160
        frame False {
          w169 = TRUE  # Loop
          n53 = Bundle By Name(cluster=T1 {"AlliGator Q Event"=enum."GUI:Toggle Playback or Loop", "Data"=variant} ("element"), "Data"=w169) -> (w170:T1)
          n54 = Build Array(w170) -> (w168:T1[])
        }
        frame True {
          n55 = global write "AlliGator Abort.vi" "Abort?"(w172) -> ()
        }
      }
      n56 = Merge Errors(w156, w158) -> (w157:errorcluster)
    }
    frame "---- Help ----" {
    }
    frame "About AlliGator" {
      n57 = Bundle By Name(cluster=T3 {"AlliGator Windows"=enum."AlliGator Window", "Open Window Options"={"Bring To Front (T)"=FALSE, "Start Hidden? (F)"=FALSE, "Activate? (T)"=FALSE}} ("output cluster"), "AlliGator Windows"=AlliGator_Windows_List."About Window", "Open Window Options.Bring To Front (T)"=TRUE, "Open Window Options.Start Hidden? (F)"=TRUE ("Start Hidden? (F)"), "Open Window Options.Activate? (T)"=TRUE) -> (w183:T3)
      n58 = Bundle By Name(cluster=T1 {"AlliGator Q Event"=enum."GUI:Open Window", "Data"=variant}, "Data"=w183) -> (w182:T1)
      n59 = Build Array(w182) -> (w176:T1[])
    }
    frame "Check for Update" {
      n60 = vi-ref "AlliGator GUI.lvlib:AlliGator Check Version.vi"() -> (w195:refnum<vi>)
      n61 = property class="VI"(reference=w195, error in=w190) -> (reference out=w186:refnum<vi>, error out=w187:errorcluster, "Path"=w194:path)
      n62 = Close Reference(reference=w186, error in (no error)=w187) -> (error out=w185:errorcluster)
      n63 = call "Run Vi.vi"("Bring To Front (T)"=FALSE, "VI Path"=w194, "error in (no error)"=w185, "Start Hidden? (F)"=TRUE, "Activate? (T)"=FALSE) -> ("error out"=w191:errorcluster)  [unwired: 3 in, 1 out]
    }
    frame "Manual" {
      n64 = call-poly <vilib>:"Open URL in Default Browser.vi"("error in (no error)"=w196, "URL"="https://alligator-distribution.readthedocs.io/") -> ("error out"=w197:errorcluster)  [unwired: 4 in, 1 out]
    }
  }
  "Error Out" <- w3
  "Message" <- w5
  "AlliGator Actions" <- w2
  "Window opened?" <- w1
